vi "Deposit.vi"(8 "error in (no error)":errorcluster, 11 "ATM Controller in":refnum<class "ATM Controller.lvclass">) -> (0 "error out":errorcluster, 3 "ATM Controller out":refnum<class "ATM Controller.lvclass">)   [LabVIEW 2019, in "ATM Controller.lvlib" / "ATM Controller.lvclass"]
uses:
  ATM Controller.lvclass
  State -Enum.ctl
  ATM Controller.lvclass/ATM Controller.ctl
  Simulated Configuration Database Actor/Configuration Database Actor Messages/Write Record Msg/Write Record Msg.lvclass/Write Record Msg.ctl
  <vilib>/ActorFramework/Message Enqueuer/Message Enqueuer.lvclass/Message Enqueuer.ctl
  <vilib>/ActorFramework/Message Enqueuer/Enqueue.vi
  Simulated Configuration Database Actor/Configuration Database Actor Messages/Write Record Msg/Write Record Msg.lvclass
  C:/Program Files (x86)/National Instruments/LabVIEW 2019/vi.lib/ActorFramework/Message/Message.lvclass
  <vilib>/ActorFramework/Message Priority Queue/Priority Enqueue.vi
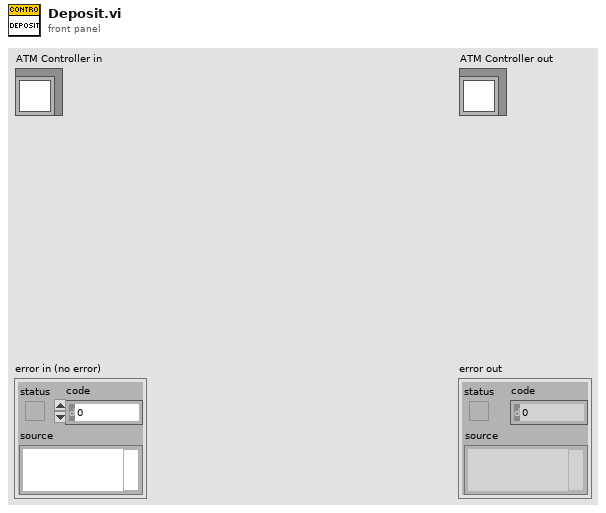
[diagram p1: front panel]
types:
  T1 = typedef "ATM Controller.lvlib/ATM Controller.lvclass/State -Enum.ctl" = enum16{"Inital", "Idle", "Login", "Balance Inquiry", "Deposit", "Withdrawal", "Fast Cash", "Terminate"}
  T2 = typedef "Configuration Database Actor.lvlib/Configuration Database Actor.lvclass/Records -cluster.ctl" = cluster{"Account Number":i32, "First Name":string, "Last Name":string, "Balance":i32}
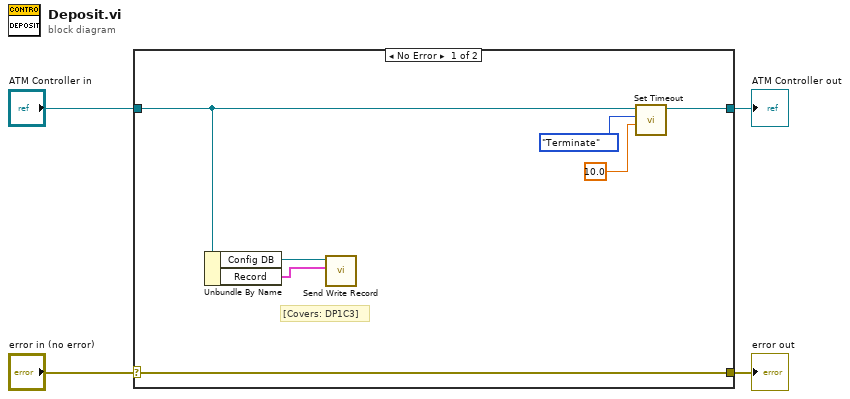
[diagram p0: block diagram]
diagram:
  n1 = case shown="No Error" "error in (no error)" {
    selector: "error in (no error)" -> [w11 w13]
    tunnel: [w11 w13] -> w3
    tunnel: [w10 w12] -> w1
    tunnel: "ATM Controller in" -> [w6 w12]
    frame No Error {
      # "[Covers: DP1C3]"
      n2 = Unbundle By Name(w6) -> ("Config DB"=w7:refnum<class "Message Enqueuer.lvclass">, "Record"=w5:T2)
      n3 = call "Send Write Record.vi"("Record"=w5, "Message Enqueuer"=w7) -> ()  [unwired: 8 in, 2 out]
      n4 = call "Set Timeout.vi"("Target Time"=10.0, "State"=State_-Enum."Terminate", "ATM Controller in"=w6) -> ("ATM Controller out"=w10:refnum<class "ATM Controller.lvclass">)  [unwired: 7 in, 1 out]
    }
    frame Error {
    }
  }
  "error out" <- w3
  "ATM Controller out" <- w1
